vi "Program Synth.vi"(8 "error in (no error)":errorcluster, 11 "NHMFL Synthesizer in":refnum<class "NHMFL Synthesizer.lvclass">) -> (0 "error out":errorcluster, 3 "NHMFL Synthesizer out":refnum<class "NHMFL Synthesizer.lvclass">)   [LabVIEW 2016, in "NHMFL Synthesizer.lvclass"]
uses:
  NHMFL Synthesizer.lvclass
  C:/Program Files/National Instruments/LabVIEW 2016/vi.lib/ActorFramework/Actor/Actor.lvclass
  <vilib>/ActorFramework/Actor/Actor.lvclass/Actor.ctl
  NHMFL Synthesizer.lvclass/NHMFL Synthesizer.ctl
  Template Module Messages/Write FP Control Msg/Write FP Control Msg.lvclass
  C:/Program Files/National Instruments/LabVIEW 2016/vi.lib/ActorFramework/Message/Message.lvclass
  Template Module Messages/Write FP Control Msg/Write FP Control Msg.lvclass/Write FP Control Msg.ctl
  Template Module Messages/Message Nested Object Msg/Message Nested Object Msg.lvclass/Message Nested Object Msg.ctl
  <vilib>/ActorFramework/Message Enqueuer/Message Enqueuer.lvclass/Message Enqueuer.ctl
  Template Module Messages/Write FP Control Msg/Write Field name.vi
  Template Module Messages/Write FP Control Msg/Write Control Value.vi
  Template Module Messages/Write FP Control Msg/Write Control Name.vi
  <vilib>/ActorFramework/Message Enqueuer/Enqueue.vi
  Template Module Messages/Message Nested Object Msg/Message Nested Object Msg.lvclass
  Read NHMFL Synthesizer Configuration.vi
  <vilib>/ActorFramework/Message Priority Queue/Priority Enqueue.vi
  <vilib>/ActorFramework/Actor/Actor.lvclass
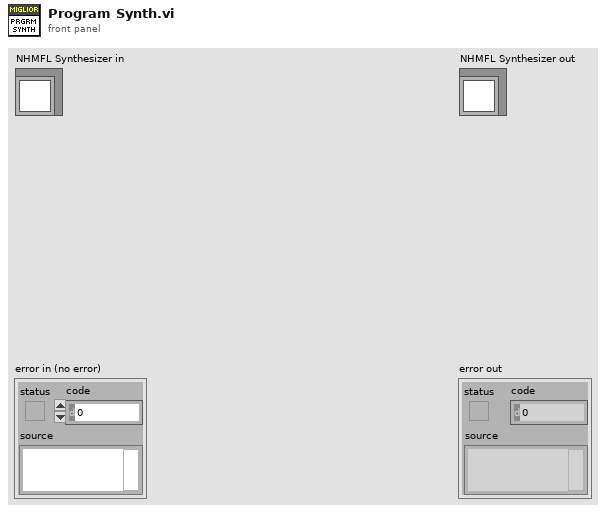
[diagram p1: front panel]
types:
  T1 = typedef "NHMFL Synthesizer Configuration.ctl" = cluster{"DAQmx Device":tag, "Variable amplitude frequency":dbl, "Fixed amplitude frequency":dbl, "Amplitude":dbl, "Clock multiplier":i32, "Channel names (variable F)":string[], "Channel names (fixed F)":string[], "Group":string, "Auto-update other modules":bool, "Recorder module":string, "Lock-in module ":string}
  T2 = typedef "Lockin Parameters.ctl" = cluster{"Frequency":dbl, "Phase":dbl, "Syncronous":bool, "Points per sine wave":i32, "DDS":bool, "Frequency word":u32, "Phase word":u32, "DDS modulus":i64, "DDS clock":dbl}
  T3 = typedef "Actual settings.ctl" = cluster{"Clock/F1":ext, "Clock/F2":ext, "F1":ext, "F2":ext, "Clock":ext}
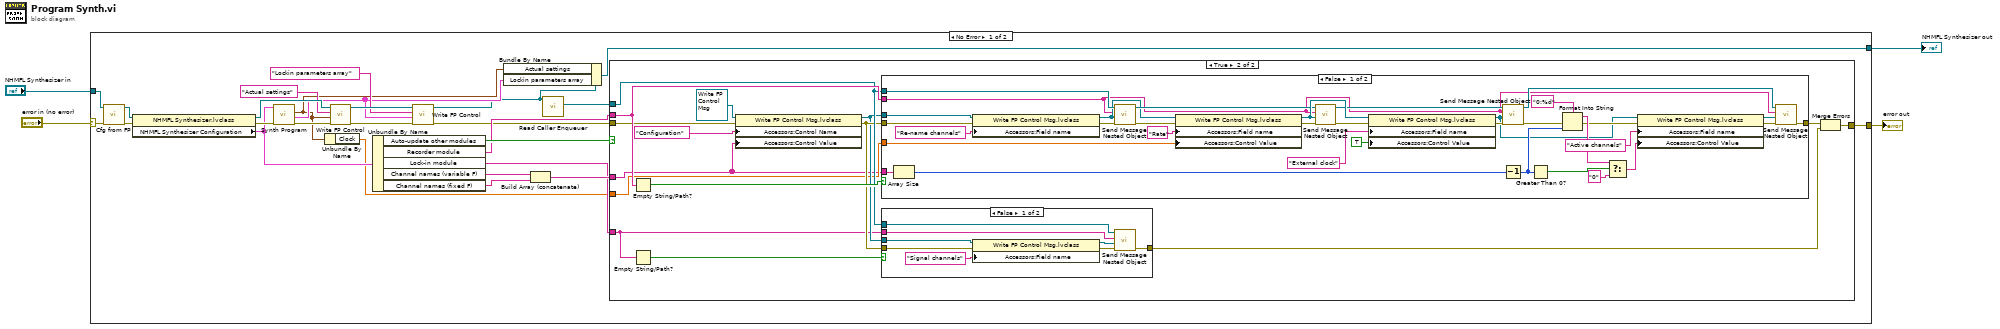
[diagram p0: block diagram]
diagram:
  n1 = case shown="No Error" "error in (no error)" {
    selector: "error in (no error)" -> [w25 w92]
    tunnel: [w7 w92] -> w3
    tunnel: [w29 w91] -> w1
    tunnel: "NHMFL Synthesizer in" -> [w22 w91]
    frame No Error {
      n2 = call-dynamic "Cfg from FP.vi"("error in (no error)"=w25, "Measure Object in"=w22) -> ("error out"=w24:errorcluster, "Measure Object out"=w30:refnum<class "NHMFL Synthesizer.lvclass">)  [unwired: 8 in]
      n3 = property class="NHMFL Synthesizer.lvclass"(reference=w30, error in=w24) -> (reference out=w27:refnum<class "NHMFL Synthesizer.lvclass">, error out=w28:errorcluster, "NHMFL Synthesizer Configuration"=w17:T1)
      n4 = call "Synth Program.vi"("Error In"=w28, "User configuration"=w17) -> ("Error Out"=w23:errorcluster, "Lockin parameters array"=w18:T2[], "Actual ratios"=w6:T3)  [unwired: 6 in, 1 out]
      n5 = Unbundle By Name(w6) -> ("Clock"=w5:ext)
      n6 = call-dynamic "Write FP Control.vi"("error in (no error)"=w23, "Control Value"=w6, "Control Name"="Actual settings", "Measure Object in"=w27) -> ("error out"=w20:errorcluster, "Measure Object out"=w21:refnum<class "NHMFL Synthesizer.lvclass">)  [unwired: 6 in]
      n7 = Unbundle By Name(w17) -> ("Auto-update other modules"=w16:bool, "Recorder module"=w15:string, "Lock-in module"=w8:string, "Channel names (variable F)"=w11:string[], "Channel names (fixed F)"=w10:string[])
      n8 = call-dynamic "Write FP Control.vi"("error in (no error)"=w20, "Control Value"=w18, "Control Name"="Lockin parameters array", "Measure Object in"=w21) -> ("error out"=w12:errorcluster, "Measure Object out"=w14:refnum<class "NHMFL Synthesizer.lvclass">)  [unwired: 6 in]
      n9 = Bundle By Name(cluster=w14, "Actual settings"=w6, "Lockin parameters array"=w18) -> (w29:refnum<class "NHMFL Synthesizer.lvclass">)
      n10 = Build Array (concatenate)(w11, w10) -> (w9:string[])
      n11 = call <vilib>:"Read Caller Enqueuer.vi"("Actor"=w14) -> ("Caller Enqueuer"=w13:refnum<class "Message Enqueuer.lvclass">)  [unwired: 10 in]
      n12 = case shown="True" w16 {
        tunnel: w15 -> [_ w45]
        tunnel: w13 -> [_ w40]
        tunnel: w12 -> [w31 w43]
        tunnel: w9 -> [_ w32]
        tunnel: w8 -> [_ w37]
        tunnel: [w31 w35] -> w7
        tunnel: w5 -> [_ w33]
        frame False {
        }
        frame True {
          n13 = Empty String/Path?(string/path=w45) -> (empty?=w46:bool)
          n14 = Empty String/Path?(string/path=w37) -> (empty?=w41:bool)
          n15 = property class="Write FP Control Msg.lvclass"(reference=refnum<class "Write FP Control Msg.lvclass"> refnum ("Write FP Control Msg.lvclass"), error in=w43, "Accessors:Control Name"="Configuration", "Accessors:Control Value"=w32) -> (reference out=w38:refnum<class "Write FP Control Msg.lvclass">, error out=w39:errorcluster)
          n16 = case shown="False" w46 {
            tunnel: w40 -> [w89 _]
            tunnel: w45 -> [w68 _]
            tunnel: w39 -> [w87 w90]
            tunnel: w38 -> [w88 _]
            tunnel: [w57 w90] -> w36
            tunnel: w33 -> [w74 _]
            tunnel: w32 -> [w67 _]
            frame False {
              n17 = Array Size(array=w67) -> (size(s)=w64:i32)
              n18 = property class="Write FP Control Msg.lvclass"(reference=w88, error in=w87, "Accessors:Field name"="Re-name channels" ("Field name")) -> (reference out=w75:refnum<class "Write FP Control Msg.lvclass">, error out=w85:errorcluster)
              n19 = call "Send Message Nested Object.vi"("error in (no error)"=w85, "Message"=w75, "Name"=w68, "Message Enqueuer"=w89) -> ("error out"=w76:errorcluster, "Message Enqueuer out"=w77:refnum<class "Message Enqueuer.lvclass">)  [unwired: 6 in]
              n20 = property class="Write FP Control Msg.lvclass"(reference=w75, error in=w76, "Accessors:Field name"="Rate" ("Field name"), "Accessors:Control Value"=w74) -> (reference out=w84:refnum<class "Write FP Control Msg.lvclass">, error out=w80:errorcluster)
              n21 = call "Send Message Nested Object.vi"("error in (no error)"=w80, "Message"=w84, "Name"=w68, "Message Enqueuer"=w77) -> ("error out"=w81:errorcluster, "Message Enqueuer out"=w82:refnum<class "Message Enqueuer.lvclass">)  [unwired: 6 in]
              n22 = property class="Write FP Control Msg.lvclass"(reference=w84, error in=w81, "Accessors:Field name"="External clock" ("Field name"), "Accessors:Control Value"=TRUE) -> (reference out=w56:refnum<class "Write FP Control Msg.lvclass">, error out=w83:errorcluster)
              n23 = call "Send Message Nested Object.vi"("error in (no error)"=w83, "Message"=w56, "Name"=w68, "Message Enqueuer"=w82) -> ("error out"=w66:errorcluster, "Message Enqueuer out"=w69:refnum<class "Message Enqueuer.lvclass">)  [unwired: 6 in]
              n24 = Decrement(x=w64) -> (x-1=w63:i32)
              n25 = Greater Than 0?(x=w63) -> (x > 0?=w62:bool)
              n26 = Format Into String(format string="0:%d", error in=w66, w63) -> (resulting string=w61:string, error out=w58:errorcluster)  [unwired: 1 in]
              n27 = Select(t=w61, s=w62, f="0") -> (s? t:f=w59:string)
              n28 = property class="Write FP Control Msg.lvclass"(reference=w56, error in=w58, "Accessors:Field name"="Active channels" ("Field name"), "Accessors:Control Value"=w59) -> (reference out=w71:refnum<class "Write FP Control Msg.lvclass">, error out=w72:errorcluster)
              n29 = call "Send Message Nested Object.vi"("error in (no error)"=w72, "Message"=w71, "Name"=w68, "Message Enqueuer"=w69) -> ("error out"=w57:errorcluster)  [unwired: 6 in, 1 out]
            }
            frame True {
            }
          }
          n30 = case shown="False" w41 {
            tunnel: w40 -> [w54 _]
            tunnel: w37 -> [w48 _]
            tunnel: w39 -> [w52 w55]
            tunnel: w38 -> [w53 _]
            tunnel: [w47 w55] -> w34
            frame False {
              n31 = property class="Write FP Control Msg.lvclass"(reference=w53, error in=w52, "Accessors:Field name"="Signal channels" ("Field name")) -> (reference out=w49:refnum<class "Write FP Control Msg.lvclass">, error out=w50:errorcluster)
              n32 = call "Send Message Nested Object.vi"("error in (no error)"=w50, "Message"=w49, "Name"=w48, "Message Enqueuer"=w54) -> ("error out"=w47:errorcluster)  [unwired: 6 in, 1 out]
            }
            frame True {
            }
          }
          n33 = Merge Errors(w36, w34) -> (w35:errorcluster)
        }
      }
    }
    frame Error {
    }
  }
  "error out" <- w3
  "NHMFL Synthesizer out" <- w1
